vi "GrabFrame.vi"(8 "error in (no error)":errorcluster, 10 "Image":u16[][](array[numeric]), 11 "CameraDAQ in":refnum<class "CameraDAQ.lvclass">) -> (0 "error out":errorcluster, 3 "CameraDAQ out":refnum<class "CameraDAQ.lvclass">)   [LabVIEW 2023, in "CameraDAQ.lvclass"]
uses:
  CameraDAQ.lvclass
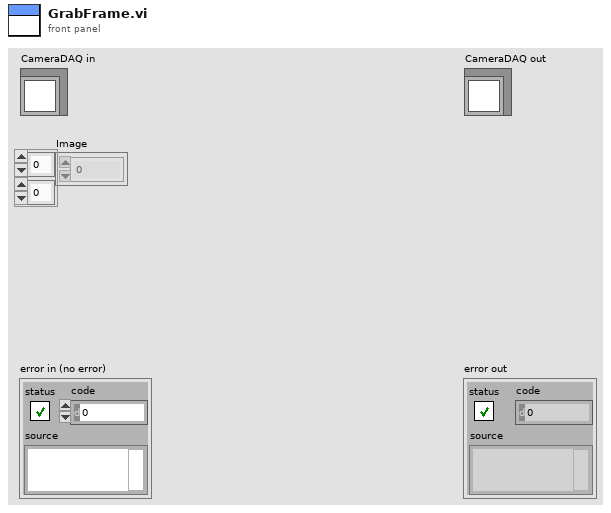
[diagram p1: front panel]
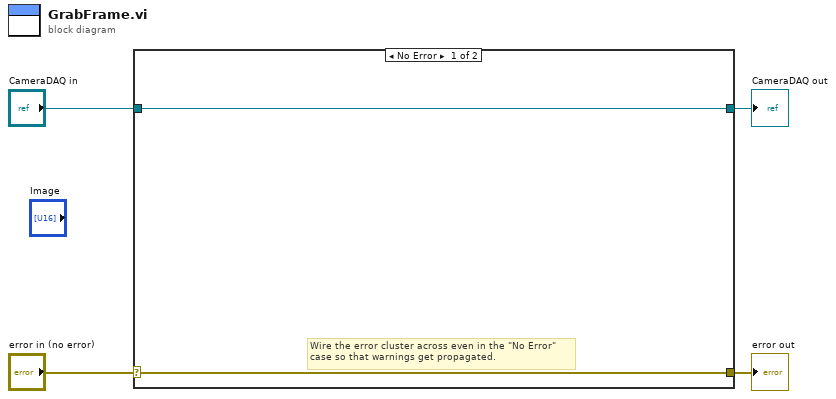
[diagram p0: block diagram]
diagram:
  n1 = case shown="No Error" "error in (no error)" {
    selector: "error in (no error)" -> [w5 w8]
    tunnel: [w5 w8] -> w3
    tunnel: [w6 w7] -> w1
    tunnel: "CameraDAQ in" -> [w6 w7]
    frame No Error {
      # "Wire the error cluster across even in the \"No Error\"\ncase so that warnings get propagated."
    }
    frame Error {
    }
  }
  "error out" <- w3
  "CameraDAQ out" <- w1
